vi "zadanie_3.vi"() -> ()   [LabVIEW 2020]
panel:
  out "string":string
  in  "String":string
  in  "stop":bool
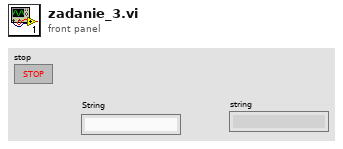
[diagram p1: front panel]
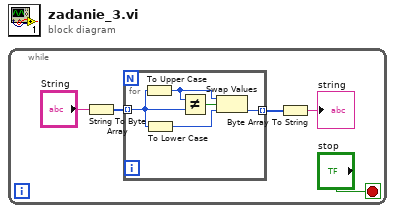
[diagram p0: block diagram]
diagram:
  n1 = while {
    stop <- "stop" stop-if-true
    n2 = String To Byte Array(string="String") -> (unsigned byte array=w3:u8[])
    n3 = for {
      tunnel: w3 -> [w10] mode=indexing
      tunnel: [w7] -> w2 mode=indexing
      n4 = To Upper Case(1:w10) -> (0:w8:u8)
      n5 = To Lower Case(string=w10) -> (all lower case string=w6:u8)
      n6 = Not Equal?(x=w8, y=w10) -> (x != y?=w9:bool)
      n7 = Swap Values(12:w8, 13:w9, 14:w6) -> (3:w7:u8)  [unwired: 1 out]
    }
    n8 = Byte Array To String(unsigned byte array=w2) -> (string=→"string":string)
  }
